vi "Get State.vi"(8 "error in (no error)":errorcluster, 11 "Tektronix MSO 6 Driver in":refnum<class "Tektronix MSO 6 Driver.lvclass">) -> (0 "error out":errorcluster, 1 "Data ready":bool, 2 "Armed":bool, 3 "Tektronix MSO 6 Driver out":refnum<class "Tektronix MSO 6 Driver.lvclass">, 4 "Availiable Samples":u32, 5 "Finished":bool)   [LabVIEW 2020, in "Tektronix MSO 6 Driver.lvclass"]
uses:
  Tektronix MSO 6 Driver.lvclass
  C:/GitHub/NHMFL_Core/Libraries/Instruments/Tektronix/Tektronix Driver/Tektronix Driver.lvclass
  <instrlib>/Tektronix MSO5X Series/Tektronix MSO5X Series.lvlib
panel:
  out "Status 3":bool
  out "Status 2":bool
  out "Status":i32(ring)=1 items=["Armed", "Auto", "Ready", "Save", "Trigger"]
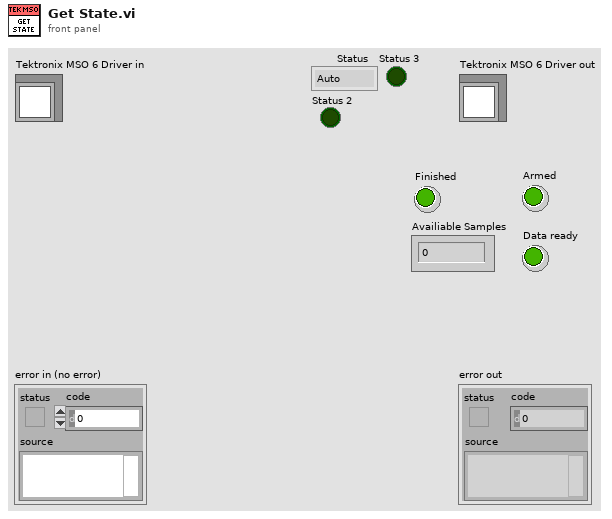
[diagram p1: front panel]
types:
  T1 = typedef "Tektronix Configuration.ctl" = cluster{"Channel":i32, "Number of averages":i32, "Input impedace":enum16{"1 M Ohm", "50 Ohm"}, "Vertical coupling":enum16{"AC", "DC", "Ground"}}
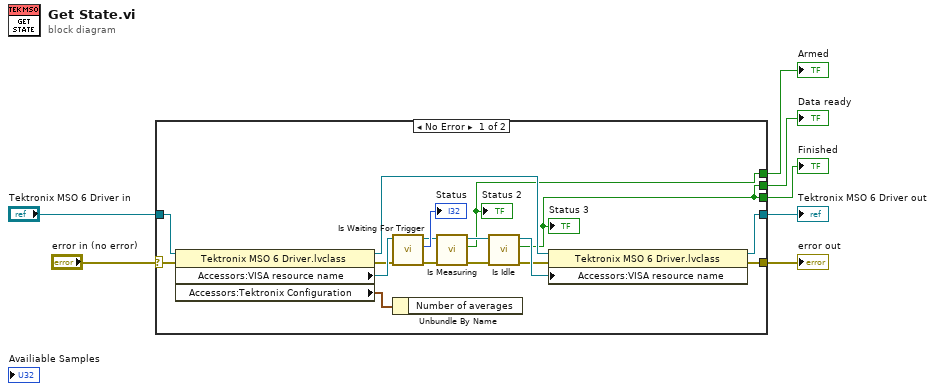
[diagram p0: block diagram]
diagram:
  n1 = case shown="No Error" "error in (no error)" {
    selector: "error in (no error)" -> [w24 w26]
    tunnel: [w21 w26] -> w2
    tunnel: [w19 w25] -> w3
    tunnel: "Tektronix MSO 6 Driver in" -> [w23 w25]
    tunnel: [w9 _] -> w5
    tunnel: [w9 _] -> w4
    tunnel: [w8 _] -> w1
    frame No Error {
      n2 = property class="Tektronix MSO 6 Driver.lvclass"(reference=w23, error in=w24) -> (reference out=w20:refnum<class "Tektronix MSO 6 Driver.lvclass">, error out=w13:errorcluster, "Accessors:VISA resource name"=w15:refnum<visa-resource-name>, "Accessors:Tektronix Configuration"=w22:T1)
      n3 = call <instrlib>:"Is Waiting For Trigger.vi"("error in (no error)"=w13, "VISA resource name"=w15) -> ("error out"=w12:errorcluster, "Status"=→"Status":i32, "VISA resource name out"=w17:refnum<visa-resource-name>)  [unwired: 7 in]
      n4 = Unbundle By Name(w22) -> ()  [unwired: 1 out]
      n5 = call <instrlib>:"Is Measuring.vi"("error in (no error)"=w12, "VISA resource name"=w17) -> ("error out"=w11:errorcluster, "Status"=w8:bool, "VISA resource name out"=w16:refnum<visa-resource-name>)  [unwired: 7 in]
      "Status 2" <- w8
      n6 = call <instrlib>:"Is Idle.vi"("error in (no error)"=w11, "VISA resource name"=w16) -> ("error out"=w10:errorcluster, "Status"=w9:bool, "VISA resource name out"=w14:refnum<visa-resource-name>)  [unwired: 7 in]
      "Status 3" <- w9
      n7 = property class="Tektronix MSO 6 Driver.lvclass"(reference=w20, error in=w10, "Accessors:VISA resource name"=w14) -> (reference out=w19:refnum<class "Tektronix MSO 6 Driver.lvclass">, error out=w21:errorcluster)
    }
    frame Error {
    }
  }
  "error out" <- w2
  "Tektronix MSO 6 Driver out" <- w3
  "Data ready" <- w5
  "Armed" <- w1
  "Finished" <- w4
